vi "Configure Air Low Temperature Limit.vi"(8 "error in (no error)":errorcluster, 9 "Air Low Temperature Limit (-150)":dbl=-150.0 min=-150.0 max=25.0 step=1.0, 11 "VISA resource name":refnum<visa-resource-name>) -> (0 "error out":errorcluster, 3 "VISA resource name out":refnum<visa-resource-name>)   [LabVIEW 2010, in "Temptronic TP04300.lvlib"]
doc: "This VI configures air low temperature limit for TP04300 instrument.\n\n<b>Air Low Temperature Limit</b> configures the minimum allowable \nair temperature in Celsius. This control accepts the minimum allowable air \ntemperature in both air and DUT modes. Out of range error will be generated \nif a setpoint exceeds this value.\n\nDefault Value: -99.9\nValid Range: -99.9 - 25.0"
uses:
  Temptronic TP04300.lvlib
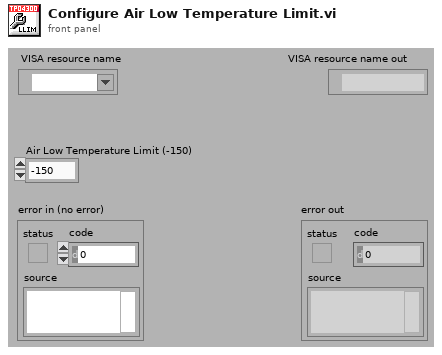
[diagram p1: front panel]
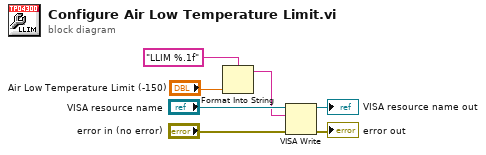
[diagram p0: block diagram]
diagram:
  n1 = Format Into String(format string="LLIM %.1f" ("multi-line string"), "Air Low Temperature Limit (-150)") -> (resulting string=w3:string)  [unwired: 2 in, 1 out]
  n2 = VISA Write(VISA resource name="VISA resource name", write buffer=w3, error in (no error)="error in (no error)") -> (VISA resource name out=→"VISA resource name out":refnum<visa-resource-name>, error out=→"error out":errorcluster)  [unwired: 1 out]
